vi "Init Parent Properties.vi"(7 "position":T1=10 items=["Open"=10, "Closed"=11], 8 "error in (no error)":errorcluster, 10 "Name":string, 11 "RelayInterface in":refnum<class "RelayInterface.lvclass">) -> (0 "error out":errorcluster, 3 "RelayInterface out":refnum<class "RelayInterface.lvclass">)   [LabVIEW 2015, in "RelayInterface.lvclass"]
doc: "This is used in a child class' New method to set the parent properties"
uses:
  RelayInterface.lvclass
  slscsl/RelayPosition.ctl
  RelayInterface.lvclass/RelayInterface.ctl
  slscsl/slscsl.lvclass
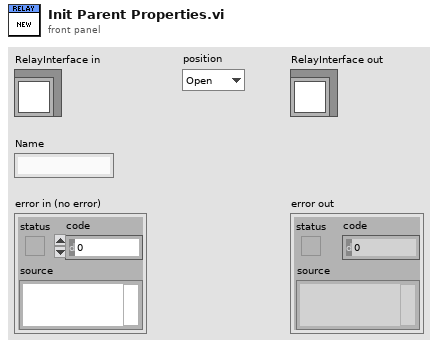
[diagram p1: front panel]
types:
  T1 = typedef "SLSC Switch.lvlib/slscsl.lvclass/RelayPosition.ctl" = i32
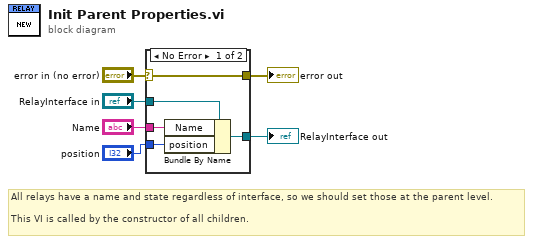
[diagram p0: block diagram]
diagram:
  # "All relays have a name and state regardless of interface, so we should set those at the parent level.\n\nThis VI is called by the constructor of all children."
  n1 = case shown="No Error" "error in (no error)" {
    selector: "error in (no error)" -> [w11 w13]
    tunnel: [w11 w13] -> w5
    tunnel: [w9 w12] -> w3
    tunnel: "RelayInterface in" -> [w10 w12]
    tunnel: "Name" -> [w8 _]
    tunnel: "position" -> [w7 _]
    frame No Error {
      n2 = Bundle By Name(cluster=w10, "Name"=w8, "position"=w7) -> (w9:refnum<class "RelayInterface.lvclass">)
    }
    frame Error {
    }
  }
  "error out" <- w5
  "RelayInterface out" <- w3
